vi "PingTestBoard.vi"(0 "COMPORT":refnum<visa-resource-name>, 5 "error in (no error)":errorcluster, 7 "Mode Select":i32(ring) items=["CW", "DYNAMIC"], 9 "Close Serial(T)":bool, 11 "ExeCommands(T)":bool) -> (2 "PyScript(path)":path=path "C:/TetraLabGUI", 12 "OK?(t)":bool=TRUE, 14 "Run_DMI(t)":bool, 15 "Run_AMInit(t)":bool, 17 "Run -dyn(t)":bool, 19 "error out":errorcluster)   [LabVIEW 2018]
uses:
  Initialize References/Sequence Globals.vi
panel:
  out "Numeric":i32
  out "standard error":string
  out "standard output":string="Server Status Ok. Received 2048 samples\r\n"
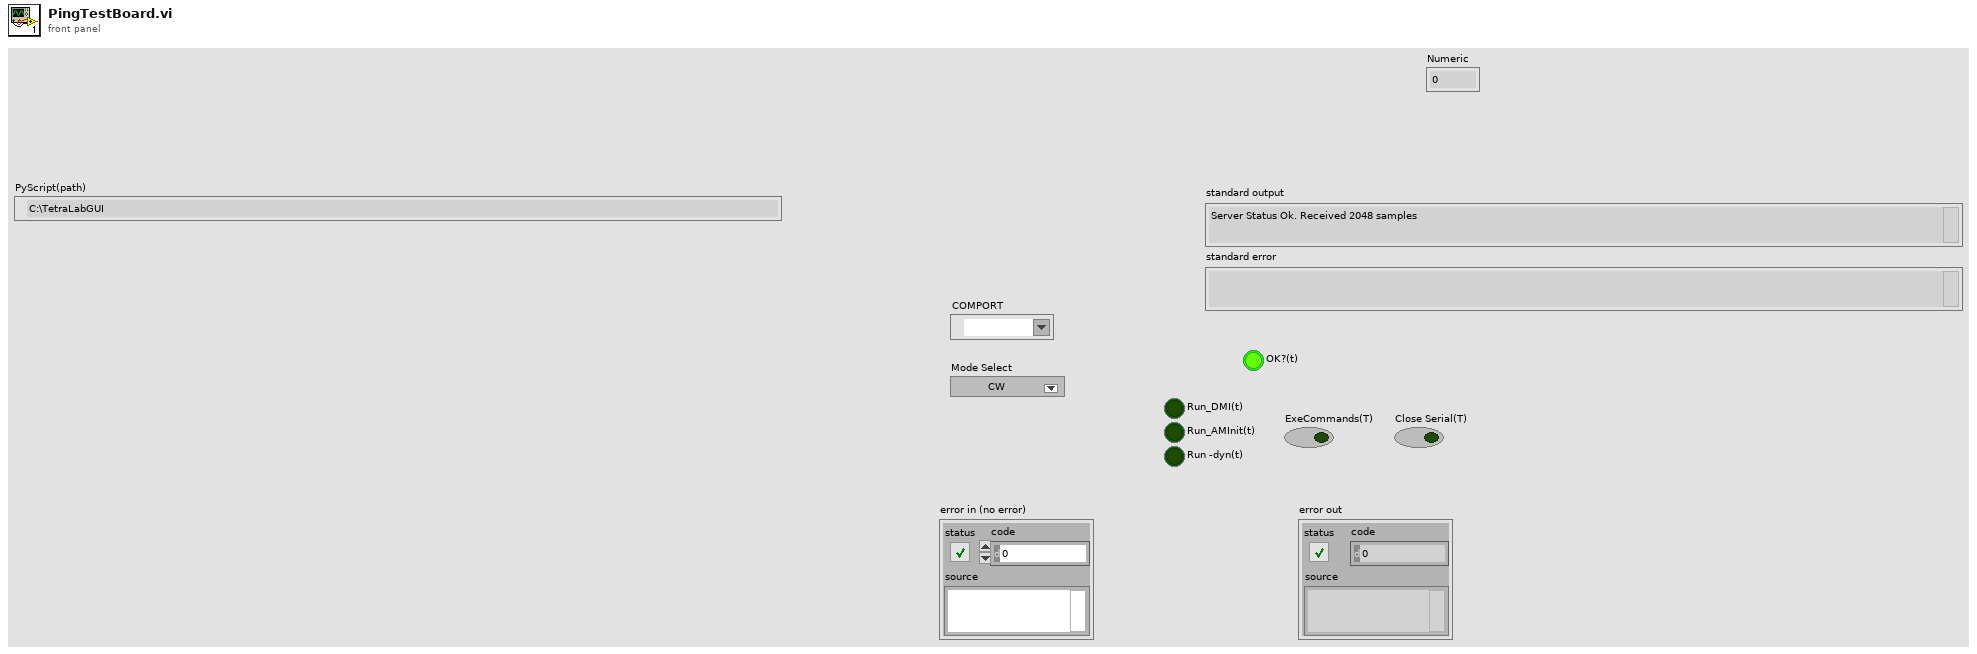
[diagram p1: front panel]
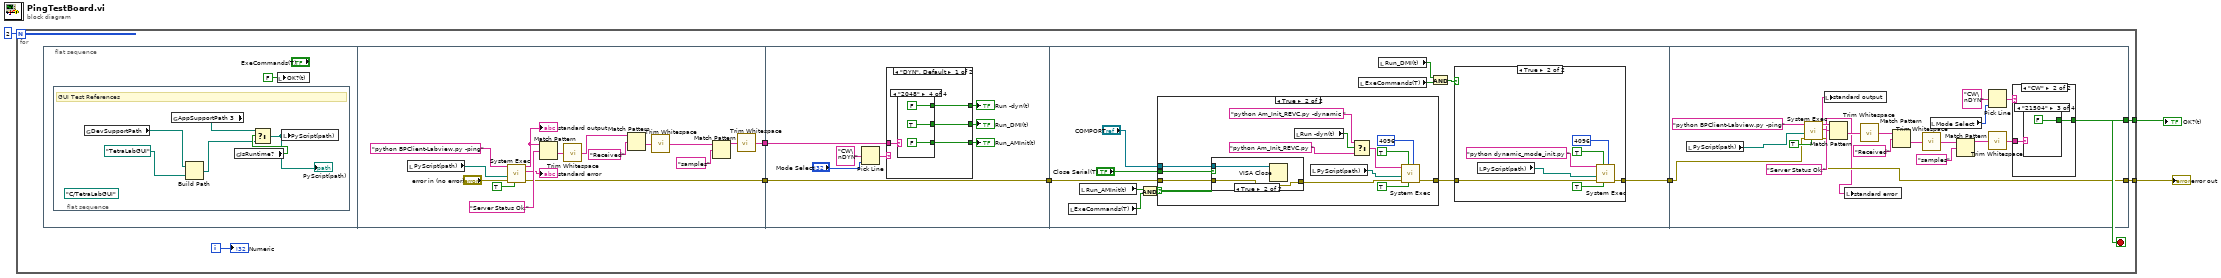
[diagram p0: block diagram]
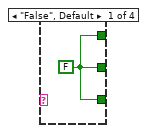
[diagram p2: hidden frame]
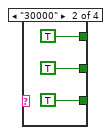
[diagram p3: hidden frame]
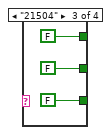
[diagram p4: hidden frame]
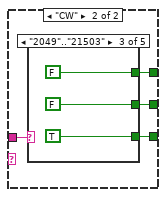
[diagram p5: hidden frame]
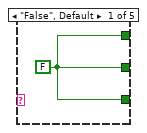
[diagram p6: hidden frame]
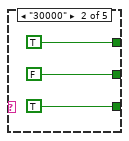
[diagram p7: hidden frame]
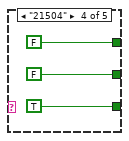
[diagram p8: hidden frame]
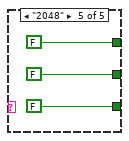
[diagram p9: hidden frame]
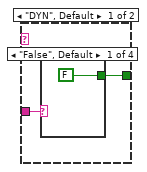
[diagram p13: hidden frame]
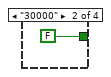
[diagram p14: hidden frame]
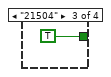
[diagram p15: hidden frame]
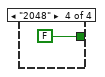
[diagram p16: hidden frame]
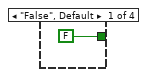
[diagram p17: hidden frame]
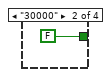
[diagram p18: hidden frame]
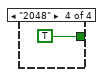
[diagram p19: hidden frame]
diagram:
  n1 = for {
    N: 2 -> [_]
    tunnel: [w6] -> w3
    tunnel: [w5] -> w2
    i -> [w4]
    stop <- w5 stop-if-true
    n2 = flat-sequence {
      tunnel: [w24] -> w10
      tunnel: [w23] -> w9
      tunnel: w10 -> [w38]
      tunnel: [w36] -> w8
      tunnel: w9 -> [w36]
      tunnel: w8 -> [w83]
      tunnel: [w81] -> w7
      tunnel: [w113] -> w6
      tunnel: w7 -> [w114]
      tunnel: [w110] -> w5
      frame #0 {
        n3 = flat-sequence {
          frame #0 {
            (unwired) path "C:/TetraLabGUI" ("PyScript(path)")
            # "GUI Test References"
            n4 = global read "Sequence Globals.vi" "DevSupportPath"() -> (w14:path)
            n5 = global read "Sequence Globals.vi" "AppSupportPath 3"() -> (w16:path)
            n6 = Build Path(base path=w14, name or relative path=path "TetraLabGUI" ("PyScript(path)")) -> (appended path=w12:path)
            n7 = global read "Sequence Globals.vi" "IsRuntime?"() -> (w17:bool)
            n8 = Select(t=w16, s=w17, f=w12) -> (s? t:f=w15:path)
            "PyScript(path)" <- w15
            n9 = local write "PyScript(path)"(w15) -> ()
          }
        }
        n10 = local write "OK?(t)"(FALSE ("OK?(t)")) -> ()
      }
      frame #1 {
        n11 = local read "PyScript(path)"() -> (w18:path)
        n12 = call <vilib>:"System Exec.vi"("run minimized? (F)"=TRUE, "error in (no error)"="error in (no error)", "working directory"=w18, "command line"="python BPClient-Labview.py -ping") -> ("error out"=w23:errorcluster, "standard error"=→"standard error":string, "standard output"=w33:string)  [unwired: 4 in, 1 out]
        "standard output" <- w33
        n13 = Match Pattern(string=w33, regular expression="Server Status Ok.") -> (after substring=w28:string)  [unwired: 1 in, 3 out]
        n14 = call <vilib>:"Trim Whitespace.vi"("string"=w28) -> ("trimmed string"=w29:string)  [unwired: 1 in]
        n15 = Match Pattern(string=w29, regular expression="Received") -> (after substring=w30:string)  [unwired: 1 in, 3 out]
        n16 = call <vilib>:"Trim Whitespace.vi"("string"=w30) -> ("trimmed string"=w32:string)  [unwired: 1 in]
        n17 = Match Pattern(string=w32, regular expression="samples") -> (before substring=w31:string)  [unwired: 1 in, 3 out]
        n18 = call <vilib>:"Trim Whitespace.vi"("string"=w31) -> ("trimmed string"=w24:string)  [unwired: 1 in]
      }
      frame #2 {
        n19 = Pick Line(multi-line string="CW\nDYN", line index="Mode Select") -> (output string=w40:string)  [unwired: 1 in]
        n20 = case shown="\"DYN\", Default" w40 {
          tunnel: w38 -> [w45 w59]
          tunnel: [w44 w58] -> w34
          tunnel: [w43 w57] -> w37
          tunnel: [w42 w56] -> w35
          frame "DYN", Default {
            n21 = case shown="\"2048\"" w45 {
              tunnel: [w46 TRUE FALSE TRUE] -> w44
              tunnel: [w46 TRUE FALSE FALSE] -> w43
              tunnel: [w46 TRUE FALSE FALSE] -> w42
              frame "False", Default {
                w46 = FALSE
              }
              frame "30000" {
              }
              frame "21504" {
              }
              frame "2048" {
              }
            }
          }
          frame "CW" {
            n22 = case shown="\"2049\"..\"21503\"" w59 {
              tunnel: [w60 FALSE FALSE FALSE FALSE] -> w58
              tunnel: [w60 TRUE TRUE TRUE FALSE] -> w57
              tunnel: [w60 TRUE FALSE FALSE FALSE] -> w56
              frame "False", Default {
                w60 = FALSE
              }
              frame "30000" {
              }
              frame "2049".."21503" {
              }
              frame "21504" {
              }
              frame "2048" {
              }
            }
          }
        }
        "Run_DMI(t)" <- w34
        "Run_AMInit(t)" <- w37
        "Run -dyn(t)" <- w35
      }
      frame #3 {
        n23 = local read "ExeCommands(T)"() -> (w75:bool)
        n24 = local read "Run_AMInit(t)"() -> (w76:bool)
        n25 = And(x=w76, y=w75) -> (x .and. y?=w80:bool)
        n26 = case shown="True" w80 {
          tunnel: w83 -> [w92 w97]
          tunnel: [w92 w102] -> w82
          tunnel: "COMPORT" -> [_ w95]
          tunnel: "Close Serial(T)" -> [_ w94]
          frame False {
          }
          frame True {
            n27 = case shown="True" w94 {
              tunnel: w97 -> [w106 w107]
              tunnel: [w106 w107] -> w96
              tunnel: w95 -> [_ w108]
              frame False {
              }
              frame True {
                n28 = VISA Close(VISA resource name=w108) -> ()  [unwired: 1 in, 1 out]
              }
            }
            n29 = local read "Run -dyn(t)"() -> (w98:bool)
            n30 = local read "PyScript(path)"() -> (w93:path)
            n31 = Select(t="python Am_Init_REVC.py -dynamic " ("command line"), s=w98, f="python Am_Init_REVC.py " ("command line")) -> (s? t:f=w101:string)
            n32 = call <vilib>:"System Exec.vi"("expected output size  (4096)"=u32 4096, "run minimized? (F)"=TRUE, "wait until completion? (T)"=TRUE, "error in (no error)"=w96, "working directory"=w93, "command line"=w101) -> ("error out"=w102:errorcluster)  [unwired: 2 in, 3 out]
          }
        }
        n33 = local read "ExeCommands(T)"() -> (w77:bool)
        n34 = local read "Run_DMI(t)"() -> (w78:bool)
        n35 = And(x=w78, y=w77) -> (x .and. y?=w79:bool)
        n36 = case shown="True" w79 {
          tunnel: [w84 w90] -> w81
          tunnel: w82 -> [w84 w87]
          frame False {
          }
          frame True {
            n37 = local read "PyScript(path)"() -> (w85:path)
            n38 = call <vilib>:"System Exec.vi"("expected output size  (4096)"=u32 4096, "run minimized? (F)"=TRUE, "wait until completion? (T)"=TRUE, "error in (no error)"=w87, "working directory"=w85, "command line"="python dynamic_mode_init.py ") -> ("error out"=w90:errorcluster)  [unwired: 2 in, 3 out]
          }
        }
      }
      frame #4 {
        n39 = local read "PyScript(path)"() -> (w109:path)
        n40 = call <vilib>:"System Exec.vi"("run minimized? (F)"=TRUE, "error in (no error)"=w114, "working directory"=w109, "command line"="python BPClient-Labview.py -ping") -> ("error out"=w113:errorcluster, "standard error"=w111:string, "standard output"=w112:string)  [unwired: 4 in, 1 out]
        n41 = local write "standard output"(w112) -> ()
        n42 = Match Pattern(string=w112, regular expression="Server Status Ok.") -> (after substring=w122:string)  [unwired: 1 in, 3 out]
        n43 = local write "standard error"(w111) -> ()
        n44 = call <vilib>:"Trim Whitespace.vi"("string"=w122) -> ("trimmed string"=w123:string)  [unwired: 1 in]
        n45 = Match Pattern(string=w123, regular expression="Received") -> (after substring=w124:string)  [unwired: 1 in, 3 out]
        n46 = call <vilib>:"Trim Whitespace.vi"("string"=w124) -> ("trimmed string"=w126:string)  [unwired: 1 in]
        n47 = local read "Mode Select"() -> (w127:i32)
        n48 = Match Pattern(string=w126, regular expression="samples") -> (before substring=w125:string)  [unwired: 1 in, 3 out]
        n49 = Pick Line(multi-line string="CW\nDYN", line index=w127) -> (output string=w121:string)  [unwired: 1 in]
        n50 = call <vilib>:"Trim Whitespace.vi"("string"=w125) -> ("trimmed string"=w128:string)  [unwired: 1 in]
        n51 = case shown="\"CW\"" w121 {
          tunnel: w128 -> [w130 w136]
          tunnel: [w129 w135] -> w110
          frame "DYN", Default {
            n52 = case shown="\"False\", Default" w130 {
              tunnel: [FALSE FALSE TRUE FALSE] -> w129
              frame "False", Default {
              }
              frame "30000" {
              }
              frame "21504" {
              }
              frame "2048" {
              }
            }
          }
          frame "CW" {
            n53 = case shown="\"21504\"" w136 {
              tunnel: [FALSE FALSE FALSE TRUE] -> w135
              frame "False", Default {
              }
              frame "30000" {
              }
              frame "21504" {
              }
              frame "2048" {
              }
            }
          }
        }
      }
    }
    "Numeric" <- w4
  }
  "error out" <- w3
  "OK?(t)" <- w2
